vi "Read Write ASCII-Unicode Text File.vi"(6 "Option":T2, 8 "error in":errorcluster, 9 "Encoding?":T1=enum."UTF-8", 10 "String In":string, 11 "file path":path) -> (0 "error out":errorcluster, 2 "String Out":string, 3 "file path Out":path)   [LabVIEW 2011]
uses:
  Unicode files/File IO/Read Write AU Text File option.ctl
  Unicode files/File IO/Text Encoding Format.ctl
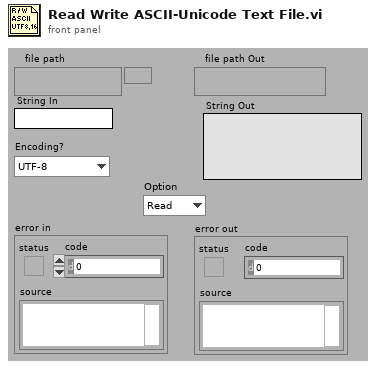
[diagram p1: front panel]
types:
  T1 = typedef "Text Encoding Format.ctl" = enum8{"ASCII", "UTF-8", "UTF-16 LE", "UTF-16 BE"}
  T2 = typedef "Read Write AU Text File option.ctl" = enum16{"Read", "Write"}
  T3 = enum16{"open", "replace", "create", "open or create", "replace or create", "replace or create with confirmation"}
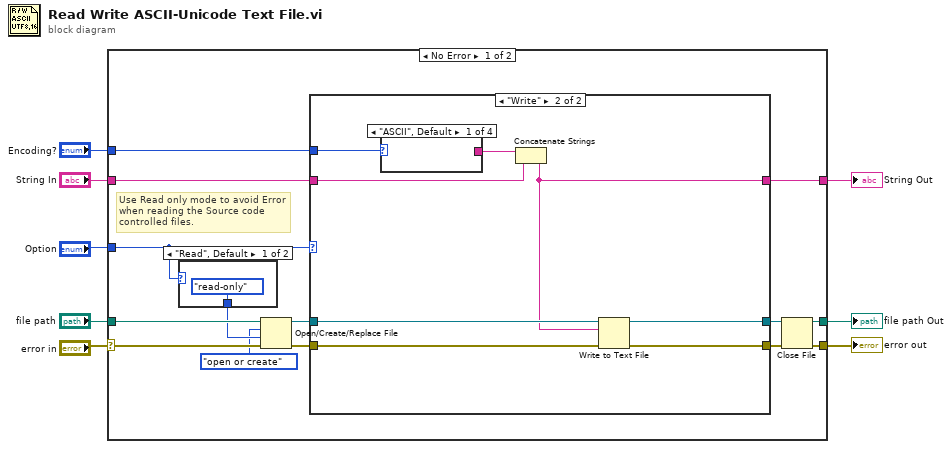
[diagram p0: block diagram]
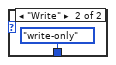
[diagram p2: hidden frame]
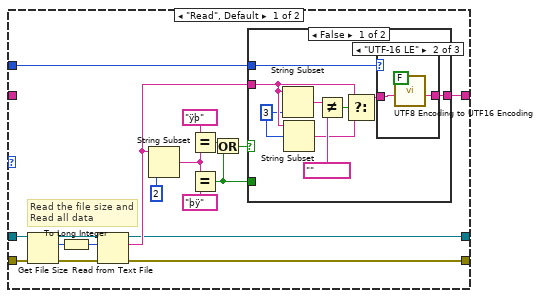
[diagram p3: hidden frame]
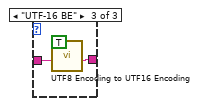
[diagram p5: hidden frame]
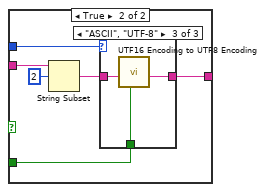
[diagram p6: hidden frame]
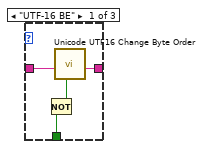
[diagram p7: hidden frame]
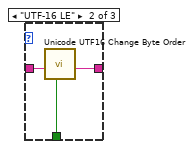
[diagram p8: hidden frame]
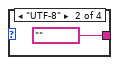
[diagram p9: hidden frame]
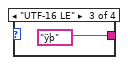
[diagram p10: hidden frame]
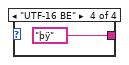
[diagram p11: hidden frame]
diagram:
  n1 = case shown="No Error" "error in" {
    selector: "error in" -> [w19 w88]
    tunnel: [w21 w88] -> w6
    tunnel: "file path" -> [w20 w87]
    tunnel: [w22 w86] -> w2
    tunnel: [w13 w87] -> w7
    tunnel: "String In" -> [w12 w86]
    tunnel: "Option" -> [w11 _]
    tunnel: "Encoding?" -> [w9 _]
    frame No Error {
      # "Use Read only mode to avoid Error \nwhen reading the Source code \ncontrolled files."
      n2 = case shown="\"Read\", Default" w11 {
        tunnel: [enum16{"read/write", "read-only", "write-only"}."read-only" ("access (0:read/write)") enum16{"read/write", "read-only", "write-only"}."write-only" ("access (0:read/write)")] -> w16
        frame "Read", Default {
        }
        frame "Write" {
        }
      }
      n3 = Open/Create/Replace File(file path (use dialog)=w20, error in=w19, operation (0:open)=T3."open or create", access (0:read/write)=w16) -> (refnum out=w15:refnum<file>, error out=w14:errorcluster)  [unwired: 2 in, 1 out]
      n4 = case shown="\"Write\"" w11 {
        tunnel: [w35 w75] -> w22
        tunnel: [w33 w80] -> w18
        tunnel: [w32 w79] -> w17
        tunnel: w15 -> [w30 w82]
        tunnel: w14 -> [w28 w81]
        tunnel: w12 -> [_ w77]
        tunnel: w9 -> [w31 w78]
        frame "Read", Default {
          # "Read the file size and \nRead all data"
          n5 = Get File Size(file=w30, error in=w28) -> (refnum out=w29:refnum<file>, size (in bytes)=w26:i64, 0:w27:errorcluster)
          n6 = To Long Integer(number=w26) -> (32bit integer=w25:i32)
          n7 = Read from Text File(file (use dialog)=w29, count=w25, error in=w27) -> (refnum out=w33:refnum<file>, text=w34:string, error out=w32:errorcluster)  [unwired: 1 in, 1 out]
          n8 = String Subset(string=w34, length (rest)=2 ("length (rest)")) -> (substring=w40:string)  [unwired: 1 in]
          n9 = Equal?(x="ÿþ" ("text 2"), y=w40) -> (x = y?=w37:bool)
          n10 = Equal?(x=w40, y="þÿ" ("text 2")) -> (x = y?=w38:bool)
          n11 = Or(x=w37, y=w38) -> (x .or. y?=w36:bool)
          n12 = case shown="False" w36 {
            tunnel: w34 -> [w47 w63]
            tunnel: [w44 w62] -> w35
            tunnel: w38 -> [_ w60]
            tunnel: w31 -> [w45 w59]
            frame False {
              w46 = 3 ("offset (0)")
              n13 = String Subset(string=w47, length (rest)=w46) -> (substring=w50:string)  [unwired: 1 in]
              n14 = String Subset(string=w47, offset (0)=w46) -> (substring=w48:string)  [unwired: 1 out]
              n15 = Not Equal?(x=w50, y="﻿" ("text 2")) -> (x != y?=w49:bool)
              n16 = Select(t=w47, s=w49, f=w48) -> (s? t:f=w43:string)
              n17 = case shown="\"UTF-16 LE\"" w45 {
                tunnel: [w52 w54 w57] -> w44
                tunnel: w43 -> [w52 w55 w58]
                frame "ASCII", "UTF-8" {
                }
                frame "UTF-16 LE" {
                  n18 = call "UTF8 Encoding to UTF16 Encoding.vi"("Big Endian?"=FALSE, "UTF-8 String"=w55) -> ("UTF-16 String"=w54:string)  [unwired: 8 in, 1 out]
                }
                frame "UTF-16 BE" {
                  n19 = call "UTF8 Encoding to UTF16 Encoding.vi"("Big Endian?"=TRUE, "UTF-8 String"=w58) -> ("UTF-16 String"=w57:string)  [unwired: 8 in, 1 out]
                }
              }
            }
            frame True {
              n20 = String Subset(string=w63, offset (0)=2) -> (substring=w61:string)  [unwired: 1 out]
              n21 = case shown="\"ASCII\", \"UTF-8\"" w59 {
                tunnel: [w66 w70 w73] -> w62
                tunnel: w61 -> [w67 w71 w74]
                tunnel: w60 -> [w68 w69 w72]
                frame "UTF-16 BE" {
                  n22 = Not(x=w68) -> (.not. x?=w65:bool)
                  n23 = call "Unicode UTF16 Change Byte Order.vi"("Change BO?"=w65, "UTF-16 String In"=w67) -> ("UTF-16 String Out"=w66:string)  [unwired: 8 in, 1 out]
                }
                frame "UTF-16 LE" {
                  n24 = call "Unicode UTF16 Change Byte Order.vi"("Change BO?"=w69, "UTF-16 String In"=w71) -> ("UTF-16 String Out"=w70:string)  [unwired: 8 in, 1 out]
                }
                frame "ASCII", "UTF-8" {
                  n25 = call "UTF16 Encoding to UTF8 Encoding.vi"("Big Endian?"=w72, "UTF-16 String"=w74) -> ("UTF-8 String"=w73:string)  [unwired: 8 in, 1 out]
                }
              }
            }
          }
        }
        frame "Write" {
          n26 = case shown="\"ASCII\", Default" w78 {
            tunnel: [_ "﻿" ("text 2") "ÿþ" ("text 2") "þÿ" ("text 2")] -> w76
            frame "ASCII", Default {
            }
            frame "UTF-8" {
            }
            frame "UTF-16 LE" {
            }
            frame "UTF-16 BE" {
            }
          }
          n27 = Concatenate Strings(w76, w77) -> (w75:string)
          n28 = Write to Text File(file (use dialog)=w82, text=w75, error in=w81) -> (refnum out=w80:refnum<file>, error out=w79:errorcluster)  [unwired: 1 in, 1 out]
        }
      }
      n29 = Close File(refnum=w18, error in=w17) -> (path=w13:path, error out=w21:errorcluster)
    }
    frame Error {
      # "Upon Error Do Nothing"
    }
  }
  "String Out" <- w2
  "error out" <- w6
  "file path Out" <- w7
